vi "Bivariate_Gaussian.vi"(8 "correlation":dbl, 10 "B":cluster{"mean":dbl, "sd":dbl}, 11 "A":cluster{"mean":dbl, "sd":dbl}) -> ()   [LabVIEW 2017]
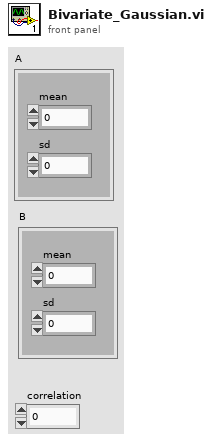
[diagram p1: front panel]
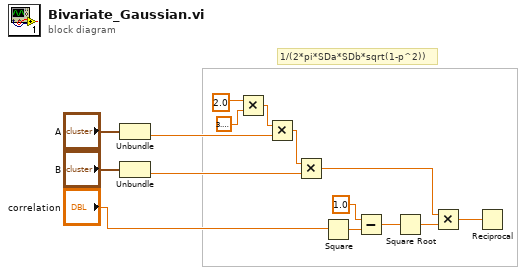
[diagram p0: block diagram]
diagram:
  # "1/(2*pi*SDa*SDb*sqrt(1-p^2))"
  n1 = Unbundle("A") -> ("sd"=w1:dbl)  [unwired: 1 out]
  n2 = Unbundle("B") -> ("sd"=w3:dbl)  [unwired: 1 out]
  n3 = Multiply(x=2.0, y=3.141592653589793) -> (x*y=w11:dbl)
  n4 = Multiply(x=w11, y=w1) -> (x*y=w10:dbl)
  n5 = Multiply(x=w10, y=w3) -> (x*y=w5:dbl)
  n6 = Square(x="correlation") -> (x^2=w9:dbl)
  n7 = Subtract(x=1.0, y=w9) -> (x-y=w7:dbl)
  n8 = Square Root(x=w7) -> (sqrt(x)=w6:dbl)
  n9 = Multiply(x=w5, y=w6) -> (x*y=w4:dbl)
  n10 = Reciprocal(x=w4) -> ()  [unwired: 1 out]
